vi "Stats Formatter.vi"(3 "Unit String":string=" us", 4 "History Data":cluster{dbl}[](array[cluster]), 5 "factor":dbl=1.0) -> (0 "Statistics String":string, 1 "Standard Deviation":dbl, 2 "Mean":dbl)   [LabVIEW 2009]
uses:
  <vilib>/Analysis/NI_AALBase.lvlib
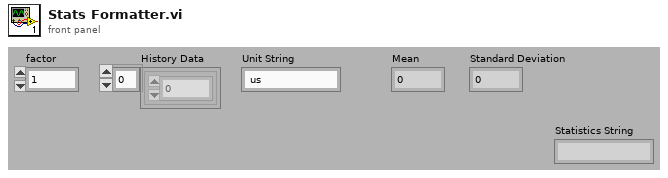
[diagram p1: front panel]
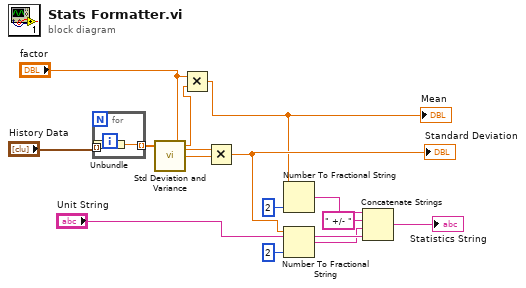
[diagram p0: block diagram]
diagram:
  n1 = for {
    tunnel: "History Data" -> [w16] mode=indexing
    tunnel: [w15] -> w2 mode=indexing
    n2 = Unbundle(w16) -> (w15:dbl)
  }
  n3 = call <vilib>:"Std Deviation and Variance.vi"("X"=w2) -> ("mean"=w3:dbl, "standard deviation"=w4:dbl)  [unwired: 1 in, 1 out]
  n4 = Multiply(x="factor", y=w3) -> (x*y=w6:dbl)
  "Mean" <- w6
  n5 = Multiply(x="factor", y=w4) -> (x*y=w8:dbl)
  "Standard Deviation" <- w8
  n6 = Number To Fractional String(number=w6, precision (6)=i16 2) -> (F-format string=w7:string)  [unwired: 2 out]
  n7 = Number To Fractional String(number=w8, precision (6)=i16 2) -> (F-format string=w9:string)  [unwired: 2 out]
  n8 = Concatenate Strings(w7, " +/- " ("string"), w9, "Unit String") -> (→"Statistics String":string)
